vi "update.vi"(7 "Pressure":dbl, 8 "error in (no error)":errorcluster, 9 "Humidity":dbl, 10 "Temperature":dbl, 11 "Display":refnum<class "DisplayBase.lvclass">) -> (0 "error out":errorcluster, 3 "Display":refnum<class "DisplayBase.lvclass">)   [LabVIEW 2020, in "DisplayBase.lvclass"]
uses:
  DisplayBase.lvclass
panel:
  # "Connector Pane"
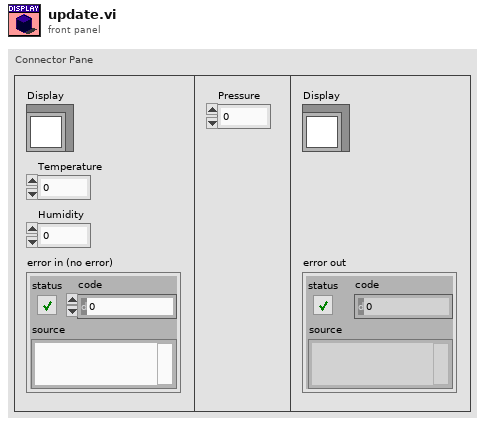
[diagram p1: front panel]
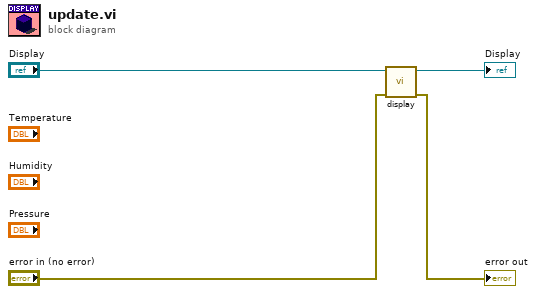
[diagram p0: block diagram]
diagram:
  n1 = call-dynamic "display.vi"("error in (no error)"="error in (no error)", "Display"="Display") -> ("error out"=→"error out":errorcluster, "CurrentConditionsDisplay.lvclass 2"=→"Display":refnum<class "DisplayBase.lvclass">)  [unwired: 8 in]
